vi "Convert BM Section From Parameter List.vi"(0 "BC Section String":string) -> (4 "BM_Messages":T1[](array[typedef]))   [LabVIEW 2011, in "AIT 1553 Custom Device.lvlib"]
uses:
  AIT 1553 Custom Device.lvlib
  Controls/1553_BM_Message.ctl
  Controls/1553 Param.ctl
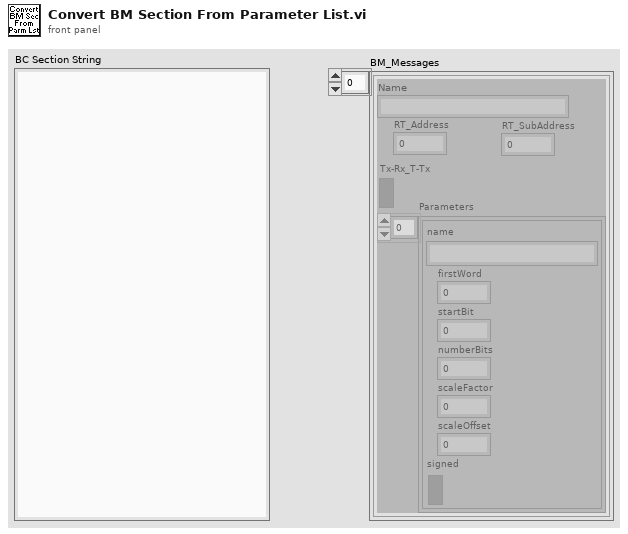
[diagram p1: front panel]
types:
  T1 = typedef "AIT 1553 Custom Device.lvlib/1553_BM_Message.ctl" = cluster{"RT_Address":u8, "RT_SubAddress":u8, "Tx-Rx_T-Tx":bool, "Parameters":T2[], "Name":string}
  T2 = typedef "AIT 1553 Custom Device.lvlib/1553 Param.ctl" = cluster{"name":string, "firstWord":i32, "startBit":i32, "numberBits":i32, "scaleFactor":dbl, "scaleOffset":dbl, "signed":bool}
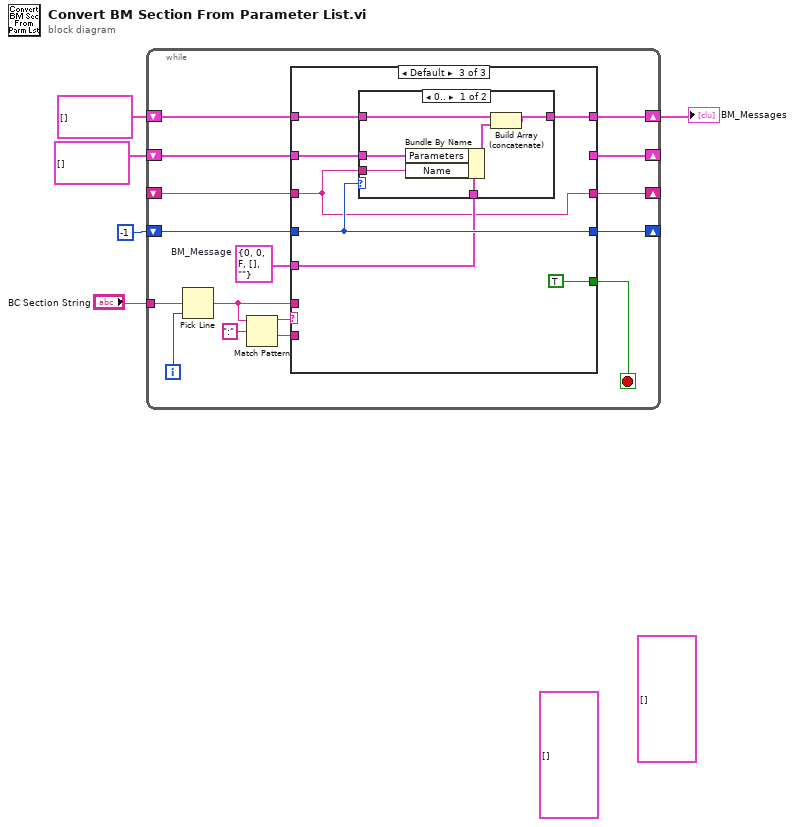
[diagram p0: block diagram]
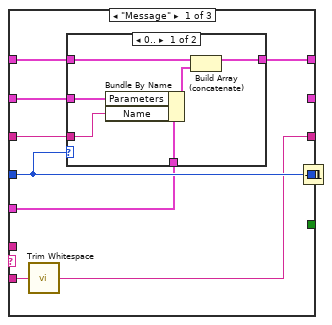
[diagram p2: hidden frame]
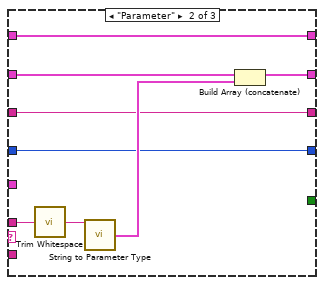
[diagram p4: hidden frame]
diagram:
  (unwired) T2[] [] ("Parameters")
  (unwired) T2[] [] ("Parameters")
  n1 = while {
    tunnel: "BC Section String" -> [w21]
    shift-right: [w18] -> w3
    shift-left: T1[] [] ("BM_Messages") -> [w19]
    shift-right: [w16] -> _
    shift-left: -1 -> [w17]
    shift-right: [w13] -> _
    shift-left: T2[] [] ("Parameters") -> [w14]
    shift-right: [w11] -> _
    shift-left: _ -> [w10]
    i -> [w8]
    stop <- w9 stop-if-true
    w6 = T1 {"RT_Address"=0, "RT_SubAddress"=0, "Tx-Rx_T-Tx"=FALSE, "Parameters"=[], "Name"=""}  # BM_Message
    n2 = Pick Line(multi-line string=w21, line index=w8) -> (output string=w15:string)  [unwired: 1 in]
    n3 = Match Pattern(string=w15, regular expression=":") -> (before substring=w7:string, after substring=w12:string)  [unwired: 1 in, 2 out]
    n4 = case shown="Default" w7 {
      tunnel: w6 -> [w23 _ w49]
      tunnel: w19 -> [w27 w44 w52]
      tunnel: [w25 w44 w48] -> w18
      tunnel: w17 -> [w28 w40 w50]
      tunnel: [w30 w40 w50] -> w16
      tunnel: w15 -> [_ w45 _]
      tunnel: w14 -> [w22 w43 w51]
      tunnel: [_ w42 _] -> w13
      tunnel: w12 -> [w29 _ _]
      tunnel: [w26 w38 w46] -> w11
      tunnel: w10 -> [w24 w38 w46]
      tunnel: [_ _ TRUE] -> w9
      frame "Message" {
        n5 = call <vilib>:"Trim Whitespace.vi"("string"=w29) -> ("trimmed string"=w26:string)  [unwired: 1 in]
        n6 = case shown="0.." w28 {
          tunnel: [w32 w37] -> w25
          tunnel: w27 -> [w35 w37]
          tunnel: w24 -> [w31 _]
          tunnel: w23 -> [w36 _]
          tunnel: w22 -> [w33 _]
          frame 0.. {
            n7 = Bundle By Name(cluster=w36, "Parameters"=w33, "Name"=w31) -> (w34:T1)
            n8 = Build Array (concatenate)(w35, w34) -> (w32:T1[])
          }
          frame Default {
          }
        }
        n9 = Increment(x=w28) -> (x+1=w30:i32)
      }
      frame "Parameter" {
        n10 = call <vilib>:"Trim Whitespace.vi"("string"=w45) -> ("trimmed string"=w39:string)  [unwired: 1 in]
        n11 = call "String to Parameter Type.vi"("String in"=w39) -> ("Parameter-1553"=w41:T2)  [unwired: 12 in, 2 out]
        n12 = Build Array (concatenate)(w43, w41) -> (w42:T2[])
      }
      frame Default {
        n13 = case shown="0.." w50 {
          tunnel: [w53 w59] -> w48
          tunnel: w52 -> [w56 w59]
          tunnel: w46 -> [w58 _]
          tunnel: w49 -> [w57 _]
          tunnel: w51 -> [w54 _]
          frame 0.. {
            n14 = Bundle By Name(cluster=w57, "Parameters"=w54, "Name"=w58) -> (w55:T1)
            n15 = Build Array (concatenate)(w56, w55) -> (w53:T1[])
          }
          frame Default {
          }
        }
      }
    }
  }
  "BM_Messages" <- w3
